vi "MouseMove.vi"(8 "error in":errorcluster, 10 "coords in":T1, 11 "class data in":refnum<class "Game.lvclass">) -> (0 "error out":errorcluster, 3 "class data out":refnum<class "Game.lvclass">)   [LabVIEW 2010, in "Labricks.lvlib" / "Game.lvclass"]
uses:
  Game.lvclass
  <vilib>/Utility/miscctls.llb/LVPoint32TypeDef.ctl
  Game.lvclass/Game.ctl
  Paddle_class/Paddle.lvclass
  RenderBase/SceneRoot_class/SceneRoot.lvclass
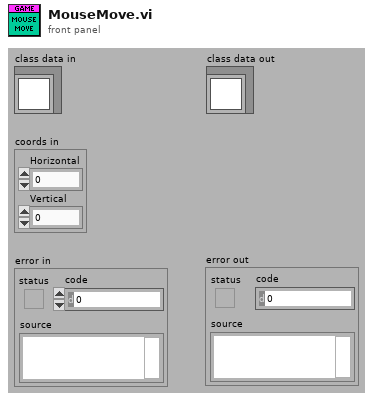
[diagram p1: front panel]
types:
  T1 = typedef "LVPoint32TypeDef.ctl" = cluster{"Horizontal":i32, "Vertical":i32}
  T2 = typedef "LV3DPointTypeDef.ctl" = cluster{"X":sgl, "Y":sgl, "Z":sgl}
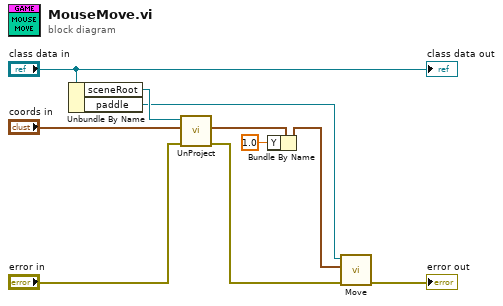
[diagram p0: block diagram]
diagram:
  n1 = Unbundle By Name("class data in") -> ("sceneRoot"=w2:refnum<class "SceneRoot.lvclass">, "paddle"=w1:refnum<class "Paddle.lvclass">)
  n2 = call "UnProject.vi"("error in"="error in", "winCoords in"="coords in", "class data in"=w2) -> ("error out"=w9:errorcluster, "sceneCoords out"=w5:T2)  [unwired: 6 in, 1 out]
  n3 = Bundle By Name(cluster=w5, "Y"=sgl 1.0) -> (w6:T2)
  n4 = call-dynamic "Move.vi"("error in (no error)"=w9, "targetCoords in"=w6, "class data in"=w1) -> ("error out"=→"error out":errorcluster)  [unwired: 7 in, 1 out]
  "class data out" <- "class data in"
